vi "saveDocument.vi"(8 "error in (no error)":errorcluster, 10 "Document Path":path, 11 "workbook in":refnum<class "workbook.lvclass">) -> (0 "error out":errorcluster, 3 "workbook out":refnum<class "workbook.lvclass">)   [LabVIEW 2017, in "Excel_Specific.lvlib" / "workbook.lvclass"]
uses:
  workbook.lvclass
  C:/Users/Neo/Desktop/Dev_Tools_BR/LabVIEW_NPOI/src/LabVIEW NPOI/NPOI_Document/npoiDocument/npoiDocument.lvclass
  workbook.lvclass/workbook.ctl
  C:/Users/Neo/Desktop/Dev_Tools_BR/LabVIEW_NPOI/src/lib/NPOI 2.1.1/NPOI.dll
  lib/NPOI 2.1.1/NPOI.dll
  NPOI_Document/npoiDocument/npoiDocument.lvclass/npoiDocument.ctl
  NPOI_Document/npoiDocument/setDocumentPath.vi
  Support/File Stream/File Stream.lvlib
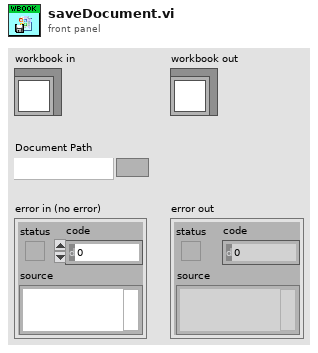
[diagram p1: front panel]
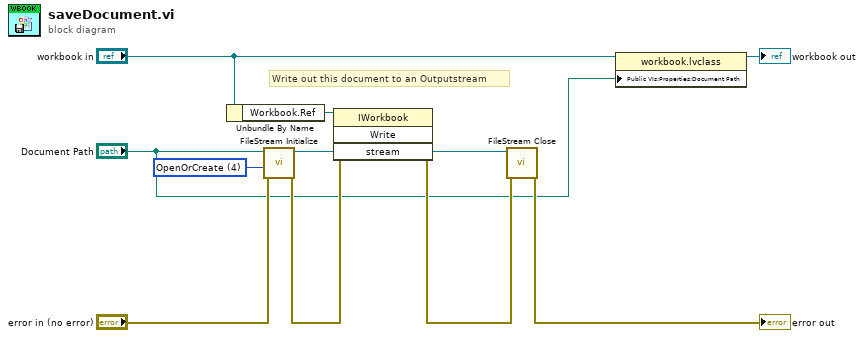
[diagram p0: block diagram]
diagram:
  w9 = 4 items=["CreateNew"=1, "Create"=2, "Open"=3, "OpenOrCreate"=4, "Truncate"=5, "Append"=6] ("operation")
  # "Write out this document to an Outputstream"
  n1 = Unbundle By Name("workbook in") -> ("Workbook.Ref"=w10:refnum<k24>)
  n2 = call "FileStream Initialize.vi"("error in (no error)"="error in (no error)", "mode"=w9, "path"="Document Path") -> ("error out"=w5:errorcluster, "new reference"=w8:refnum<k24>)  [unwired: 7 in]
  n3 = invoke class="IWorkbook" method="Write"(reference=w10, error in=w5, "stream"=w8) -> (error out=w6:errorcluster)  [unwired: 1 in, 3 out]
  n4 = call "FileStream Close.vi"("error in (no error)"=w6, "reference"=w8) -> ("error out"=→"error out":errorcluster)  [unwired: 9 in]
  n5 = property class="workbook.lvclass"(reference="workbook in", "Public VIs:Properties:Document Path"="Document Path") -> (reference out=→"workbook out":refnum<class "workbook.lvclass">)  [unwired: 1 in, 1 out]
